vi "Digitize I and Q signals.vi"(1 "Sample Frequency":u8(ring)=6 items=["4000.0", "5512.50", "6000.00", "6400.00", "8000.00", "11025.00", "12000.00", "12800.00", "16000.00", "22050.00", "24000.00", "25600.00", "32000.00", "44100.00", "48000.00", "51200.00"], 2 "total sampling time":sgl=3.0 min=0 format="%.2f", 5 "file path (dialog if empty)":path=path "d:/doppler_data") -> ()   [LabVIEW 2022 SP3]
doc: "Scanning siganls from the doppler. WITH NO DISPLAY OF DATA FROM FFT ROUTINE"
panel:
  in  "change window parameters ?":bool
  in  "stop":bool
  out "Current data file":path
  in  "?":dbl[](array[numeric])=[4000.0, 5512.5, 6000.0, 6400.0, 8000.0, 11025.0, 12000.0, 12800.0, 16000.0, 22050.0, 24000.0, 25600.0, 32000.0, 44100.0, 48000.0, 51200.0] format="%.2f"
  out "A to  D param":T1={"device (1)"=1, "channels (0)"=["0:1"], "number of samples\nto acquire"=1024, "sample rate "=6000.0, "input limits "=[{"high limit"=0.5, "low limit"=-0.5}]} {"input limits"."low limit" format="%.2f"; "input limits"."high limit" format="%.2f"; "sample rate" format="%.2f"}
  in  "digitize":bool=TRUE
  in  "A to  D param":T1={"device (1)"=1, "channels (0)"=["0:1"], "number of samples\nto acquire"=1024, "sample rate "=6000.0, "input limits "=[{"high limit"=0.5, "low limit"=-0.5}]} {"input limits"."low limit" format="%.2f"; "input limits"."high limit" format="%.2f"; "sample rate" format="%.2f"}
  # "Input Variables"
  # "Change Values"
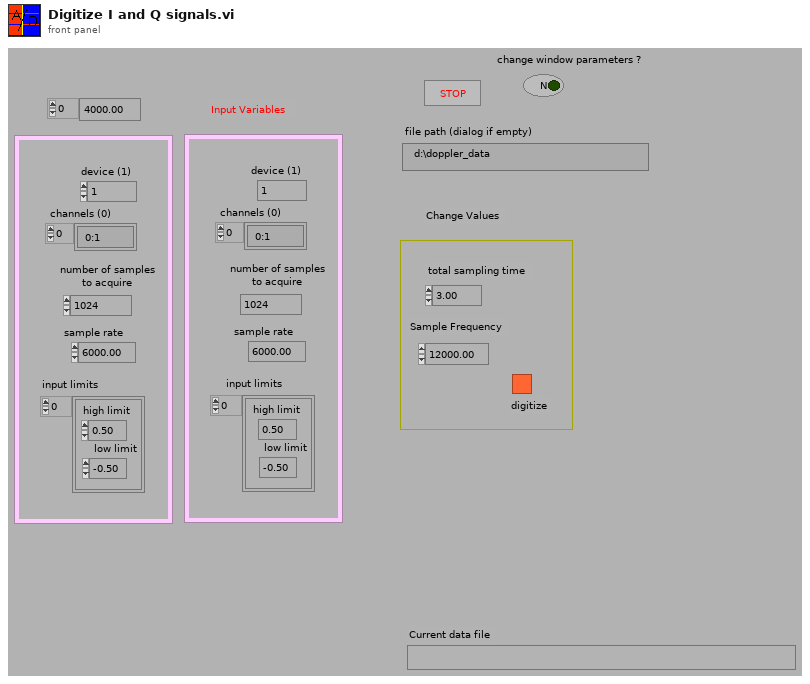
[diagram p1: front panel]
types:
  T1 = cluster{"device (1)":u8, "channels (0)":string[], "number of samples\nto acquire":u32, "sample rate ":sgl, "input limits ":cluster{"high limit":sgl, "low limit":sgl}[]}
  T2 = cluster{"number of samples\nto acquire":u32, "sample rate ":sgl, "voltage data":sgl[][]}
  T3 = cluster{"total time slices":i32, "f0":dbl, "Df":dbl, "Dt":dbl}
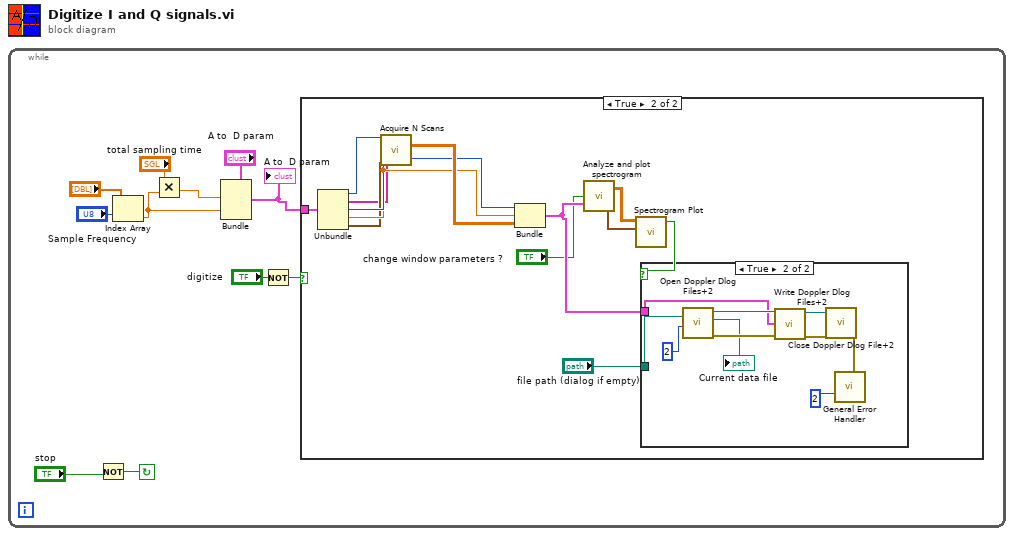
[diagram p0: block diagram]
diagram:
  n1 = while {
    stop <- w11 continue-if-true
    n2 = Not(x="stop") -> (.not. x?=w11:bool)
    n3 = Index Array(array="?", index="Sample Frequency") -> (element=w3:dbl)
    n4 = Multiply(x="total sampling time", y=w3) -> (x*y=w8:dbl)
    n5 = Bundle(cluster="A to  D param", "number of samples\nto acquire"=w8, "sample rate"=w3) -> (w9:T1)  [unwired: 3 in]
    "A to  D param" <- w9
    n6 = Not(x="digitize") -> (.not. x?=w1:bool)
    n7 = case shown="True" w1 {
      tunnel: w9 -> [_ w12]
      frame False {
      }
      frame True {
        n8 = Unbundle(w12) -> ("device (1)"=w13:u8, "channels (0)"=w14:string[], "number of samples\nto acquire"=w23:u32, "sample rate"=w22:sgl, "input limits"=w15:cluster{"high limit":sgl, "low limit":sgl}[])
        n9 = call "Acquire N Scans.vi"("device (1)"=w13, "channels (0)"=w14, "number of scans\nto acquire (1000)"=w23, "scan rate\n(1000 scans/sec)"=w22, "input limits (no change)"=w15) -> ("voltage data"=w24:sgl[][])  [unwired: 9 in, 1 out]
        n10 = Bundle("number of samples\nto acquire"=w23, "sample rate"=w22, "voltage data"=w24) -> (w20:T2)  [unwired: 1 in]
        n11 = call "Analyze and plot spectrogram .vi"("change window parameters ?"="change window parameters ?", "datalog record"=w20) -> ("Spectrogram Plotting Parameters"=w18:T3, "Spectrogram"=w19:dbl[][])  [unwired: 1 in]
        n12 = call "Spectrogram Plot.vi"("FFT{I,Q}"=w19, "Spectrogram parameters"=w18) -> ("Save data"=w16:bool)  [unwired: 6 in]
        n13 = case shown="True" w16 {
          tunnel: "file path (dialog if empty)" -> [_ w29]
          tunnel: w20 -> [_ w25]
          frame False {
          }
          frame True {
            n14 = call "Open Doppler Dlog Files+2.vi"("function (open:0)"=2, "start path  (Not A Path)"=w29) -> ("error out"=w30:errorcluster, "new file path"=→"Current data file":path, "refnum"=w27:refnum<k1>)  [unwired: 6 in, 1 out]
            n15 = call "Write Doppler Dlog Files+2.vi"("error in (no error)"=w30, "datalog record"=w25, "refnum"=w27) -> ("error out"=w34:errorcluster, "refnum"=w33:refnum<k1>)  [unwired: 6 in, 1 out]
            n16 = call "Close Doppler Dlog File+2.vi"("error in (no error)"=w34, "refnum"=w33) -> ("error out"=w31:errorcluster)  [unwired: 3 in, 2 out]
            n17 = call <vilib>:"General Error Handler.vi"("type of dialog (OK msg:1)"=2 ("continue or stop message on an error"), "error in (no error)"=w31) -> ()  [unwired: 9 in, 5 out]
          }
        }
      }
    }
  }
